vi "Quad Encoder Settings.vi"() -> ()   [LabVIEW 2020]
uses:
  Submodules/Source/Types/QuadratureEncoder.Measure.Digital.Settings.ctl
  <vilib>/rvi/Emulation/niFpgaGetClockAttributes.vi
  <vilib>/rvi/Emulation/niFpgaSctlEmulationGetInTimedLoop.vi
  <vilib>/rvi/Emulation/niFpgaEmulationReportErrorSimple.vi
  <vilib>/rvi/Emulation/niFpgaCriticalErrorInLSC.vi
  Submodules/Source/Speciality FPGA IO.lvlib
panel:
  out "Z RESET STATE":bool
  out "B RESET STATE":bool
  out "A RESET STATE":bool
  out "RESET VALUE":i32
  out "DIRECTION":u8
  in  "Quad Encoder Settings":T1
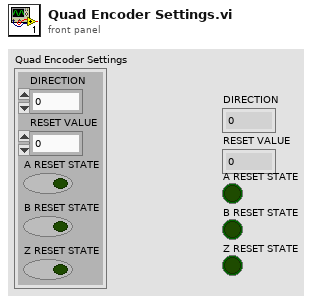
[diagram p1: front panel]
types:
  T1 = typedef "Speciality FPGA IO.lvlib/QuadratureEncoder.Measure.Digital.Settings.ctl" = cluster{"DIRECTION":u8, "RESET VALUE":i32, "A RESET STATE":bool, "B RESET STATE":bool, "Z RESET STATE":bool}
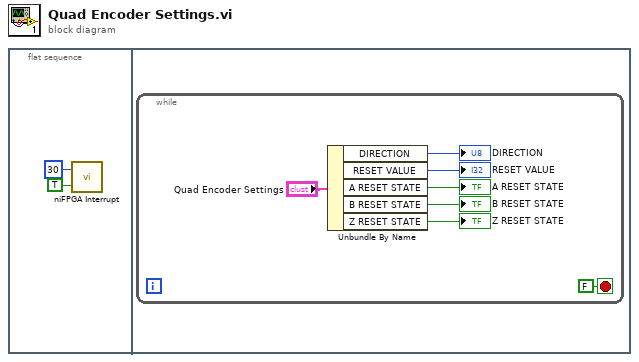
[diagram p0: block diagram]
diagram:
  n1 = flat-sequence {
    frame #0 {
      n2 = call <vilib>:"niFPGA Interrupt.vi"("Wait Until Cleared (F)"=TRUE, "IRQ Number (0)"=u8 30) -> ()  [unwired: 1 in]
    }
    frame #1 {
      n3 = while {
        stop <- FALSE stop-if-true
        n4 = Unbundle By Name("Quad Encoder Settings") -> ("DIRECTION"=→"DIRECTION":u8, "RESET VALUE"=→"RESET VALUE":i32, "A RESET STATE"=→"A RESET STATE":bool, "B RESET STATE"=→"B RESET STATE":bool, "Z RESET STATE"=→"Z RESET STATE":bool)
      }
    }
  }
